vi "Get Actual Power.vi"(8 "error in":errorcluster, 10 "?":T1, 11 "HSU MCU V2 CFG in":refnum<class "HSU MCU V2 CFG.lvclass">) -> (0 "error out":errorcluster, 1 "Torque":dbl format="%#_g Nm", 2 "Power":dbl format="%#_g W", 3 "HSU MCU V2 CFG out":refnum<class "HSU MCU V2 CFG.lvclass">)   [LabVIEW 2024, in "HSU MCU V2 CFG.lvclass"]
uses:
  HSU MCU V2 CFG.lvclass
  MCU Selector.ctl
  HSU MCU V2 CFG.lvclass/HSU MCU V2 CFG.ctl
  Protocols/ICAN/ICAN.lvclass
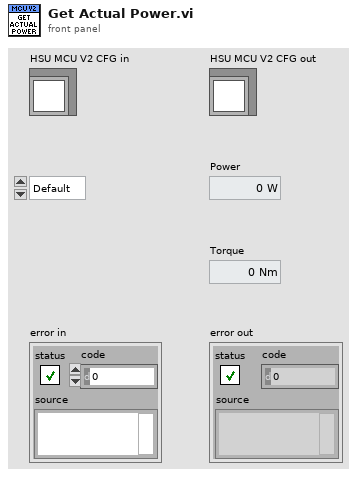
[diagram p1: front panel]
types:
  T1 = typedef "MCU Selector.ctl" = enum16{"Default", "MCU1", "MCU2", "MCU3", "MCU4", "MCU5", "MCU6", "MCU7", "MCU8", "ALL"}
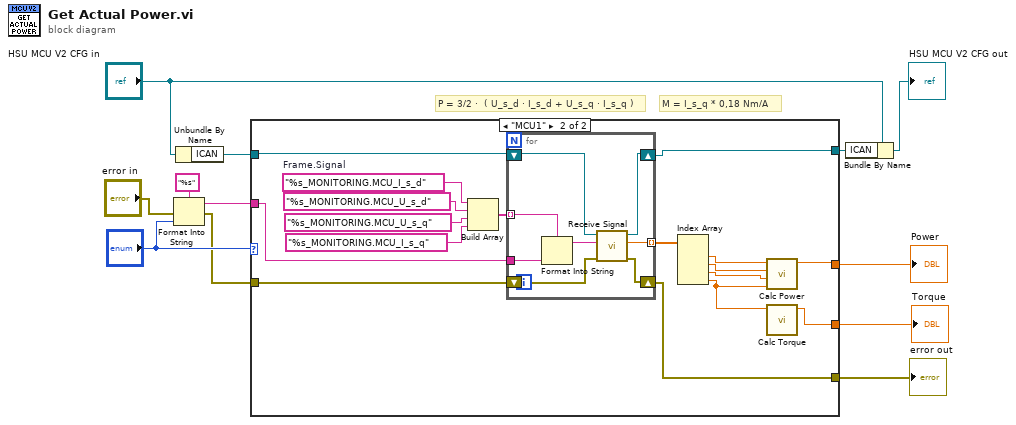
[diagram p0: block diagram]
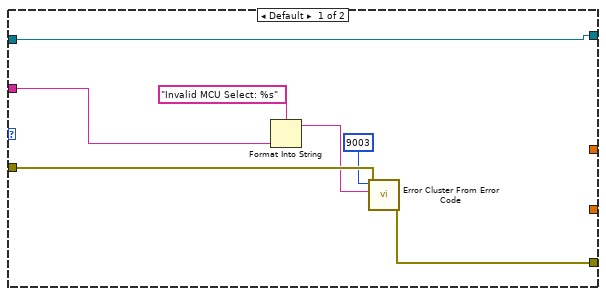
[diagram p2: hidden frame]
diagram:
  # "M = I_s_q * 0,18 Nm/A"
  # "P = 3/2 ·  ( U_s_d · I_s_d + U_s_q · I_s_q )"
  n1 = Format Into String(format string="%s", error in="error in", "?") -> (resulting string=w10:string, error out=w1:errorcluster)  [unwired: 1 in]
  n2 = Unbundle By Name("HSU MCU V2 CFG in") -> ("ICAN"=w9:refnum<class "ICAN.lvclass">)
  n3 = case shown="\"MCU1\"" "?" {
    tunnel: w1 -> [w19 w29]
    tunnel: [w18 w27] -> w7
    tunnel: w10 -> [w14 w31]
    tunnel: w9 -> [w13 w30]
    tunnel: [_ w25] -> w8
    tunnel: [w13 w26] -> w6
    tunnel: [_ w20] -> w3
    frame Default {
      n4 = Format Into String(format string="Invalid MCU Select: %s" ("error message (\"\")"), w14) -> (resulting string=w16:string)  [unwired: 2 in, 1 out]
      n5 = call <vilib>:"Error Cluster From Error Code.vi"("error in (no error)"=w19, "error message (\"\")"=w16, "error code (0)"=9003) -> ("error out"=w18:errorcluster)  [unwired: 6 in]
    }
    frame "MCU1" {
      w36 = "%s_MONITORING.MCU_I_s_d"  # Frame.Signal
      n6 = Build Array(w36, "%s_MONITORING.MCU_U_s_d" ("Frame.Signal"), "%s_MONITORING.MCU_U_s_q" ("Frame.Signal"), "%s_MONITORING.MCU_I_s_q" ("Frame.Signal")) -> (w32:string[])
      n7 = for {
        tunnel: w32 -> [w43] mode=indexing
        tunnel: w31 -> [w44]
        tunnel: [w38] -> w28 mode=indexing
        shift-right: [w39] -> w27
        shift-left: w29 -> [w40]
        shift-right: [w37] -> w26
        shift-left: w30 -> [w42]
        n8 = Format Into String(format string=w43, w44) -> (resulting string=w41:string)  [unwired: 2 in, 1 out]
        n9 = call-dynamic "Receive Signal.vi"("error in"=w40, "Frame.Signal"=w41, "ICommunicate in"=w42) -> ("error out"=w39:errorcluster, "Value"=w38:dbl, "ICommunicate out"=w37:refnum<class "ICAN.lvclass">)  [unwired: 6 in]
      }
      n10 = Index Array(array=w28) -> (element #1=w24:dbl, element #2=w23:dbl, element #3=w22:dbl, element #4=w21:dbl)  [unwired: 4 in]
      n11 = call "Calc Power.vi"("MCU_I_s_q"=w21, "MCU_U_s_q"=w22, "MCU_U_s_d"=w23, "MCU_I_s_d"=w24) -> ("Power"=w25:dbl)  [unwired: 7 in]
      n12 = call "Calc Torque.vi"("MCU_I_s_q"=w21) -> ("Torque"=w20:dbl)  [unwired: 10 in]
    }
  }
  "error out" <- w7
  "Power" <- w8
  "Torque" <- w3
  n13 = Bundle By Name(cluster="HSU MCU V2 CFG in", "ICAN"=w6) -> (→"HSU MCU V2 CFG out":refnum<class "HSU MCU V2 CFG.lvclass">)
